vi "GetLibFromProject.vi"(0 "ProjectPath":path, 1 "error in (no error)":errorcluster) -> (2 "LibraryPath":path, 3 "SingleLib?":bool, 4 "LibraryName":string, 5 "error out":errorcluster)   [LabVIEW 2009, in "HGF_VisitorGenerator.lvlib"]
doc: "Get library from given project.\nexpected is one library except the agent base lib...the one with the agent class inside"
uses:
  HGF_VisitorGenerator.lvlib
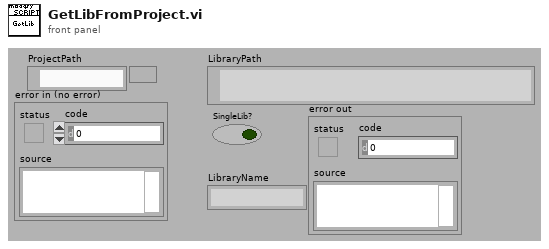
[diagram p1: front panel]
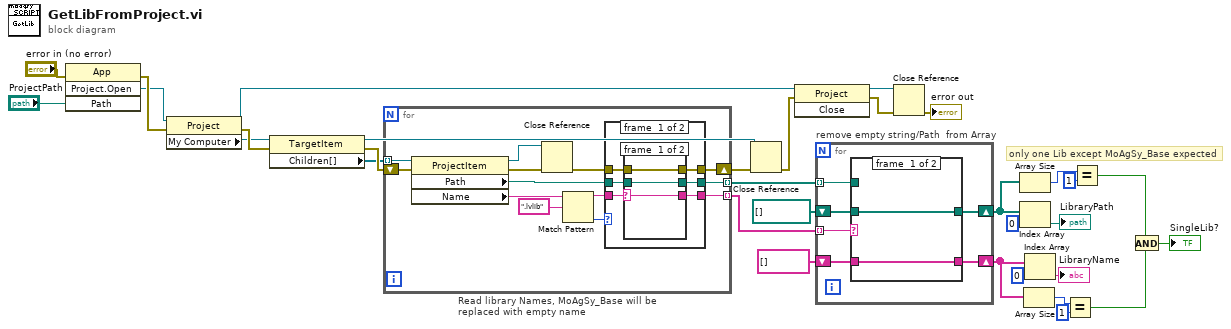
[diagram p0: block diagram]
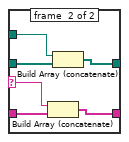
[diagram p2: hidden frame]
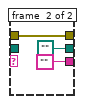
[diagram p3: hidden frame]
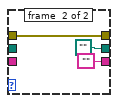
[diagram p4: hidden frame]
diagram:
  # "only one Lib except MoAgSy_Base expected"
  n1 = invoke class="App" method="Project.Open"(error in="error in (no error)", "Path"="ProjectPath") -> (error out=w13:errorcluster, "Project:Open"=w10:refnum<vi>)  [unwired: 2 in, 2 out]
  n2 = property class="Project"(reference=w10, error in=w13) -> (reference out=w11:refnum<vi>, error out=w14:errorcluster, "My Computer"=w4:refnum<vi>)
  n3 = property class="TargetItem"(reference=w4, error in=w14) -> (reference out=w3:refnum<vi>, error out=w15:errorcluster, "Children[]"=w12:refnum<vi>[])
  n4 = for "Read library Names, MoAgSy_Base will be replaced with empty name" {
    tunnel: w12 -> [w45] mode=indexing
    shift-right: [w37] -> w6
    shift-left: w15 -> [w44]
    tunnel: [w40] -> w17 mode=indexing
    tunnel: [w36] -> w16 mode=indexing
    n5 = property class="ProjectItem"(reference=w45, error in=w44) -> (reference out=w35:refnum<vi>, error out=w34:errorcluster, "Path"=w38:path, "Name"=w39:string)
    n6 = Close Reference(reference=w35, error in (no error)=w34) -> (error out=w33:errorcluster)
    n7 = Match Pattern(string=w39, regular expression=".lvlib") -> (before substring=w41:string, offset past match=w42:i32)  [unwired: 1 in, 2 out]
    n8 = case shown="Default" w42 {
      tunnel: w41 -> [w51 _]
      tunnel: [w50 ""] -> w40
      tunnel: w38 -> [w49 _]
      tunnel: w33 -> [w48 w60]
      tunnel: [w47 w60] -> w37
      tunnel: [w46 path ""] -> w36
      frame #0 {
        n9 = case shown="\"MoAgSy_Base\"" w51 {
          selector: w51 -> [w54 _]
          tunnel: [w54 ""] -> w50
          tunnel: w49 -> [w53 _]
          tunnel: w48 -> [w52 w57]
          tunnel: [w52 w57] -> w47
          tunnel: [w53 path ""] -> w46
          frame #0 {
          }
          frame #1 {
          }
        }
      }
      frame #1 {
      }
    }
  }
  n10 = Close Reference(reference=w3, error in (no error)=w6) -> (error out=w5:errorcluster)
  n11 = invoke class="Project" method="Close"(reference=w11, error in=w5) -> (reference out=w2:refnum<vi>, error out=w7:errorcluster)  [unwired: 1 in, 1 out]
  n12 = for "remove empty string/Path  from Array" {
    tunnel: w16 -> [w61] mode=indexing
    tunnel: w17 -> [w66] mode=indexing
    shift-right: [w62] -> w23
    shift-left: path[] [] -> [w63]
    shift-right: [w64] -> w24
    shift-left: string[] [] -> [w65]
    n13 = case shown="Default" w66 {
      selector: w66 -> [_ w69]
      tunnel: w65 -> [w68 w71]
      tunnel: [w68 w70] -> w64
      tunnel: w63 -> [w67 w74]
      tunnel: [w67 w73] -> w62
      tunnel: w61 -> [_ w72]
      frame #0 {
      }
      frame #1 {
        n14 = Build Array (concatenate)(w69, w71) -> (w70:string[])
        n15 = Build Array (concatenate)(w72, w74) -> (w73:path[])
      }
    }
  }
  n16 = Close Reference(reference=w2, error in (no error)=w7) -> (error out=→"error out":errorcluster)
  n17 = Array Size(array=w23) -> (size(s)=w29:i32)
  n18 = Index Array(array=w23, index=0) -> (element=→"LibraryPath":path)
  n19 = Array Size(array=w24) -> (size(s)=w26:i32)
  n20 = Index Array(array=w24, index=0) -> (element=→"LibraryName":string)
  n21 = Equal?(x=w26, y=1) -> (x = y?=w31:bool)
  n22 = Equal?(x=w29, y=1) -> (x = y?=w30:bool)
  n23 = And(x=w30, y=w31) -> (x .and. y?=→"SingleLib?":bool)
